vi "To Unix Time.vi"(0 "timestamp":timestamp) -> (2 "unix time":u32)   [LabVIEW 2013, in "libssh2.lvlib"]
doc: "Convert a LabVIEW timestamp to Unix time."
uses:
  libssh2.lvlib
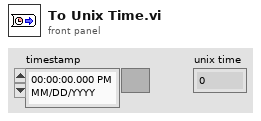
[diagram p1: front panel]
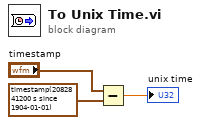
[diagram p0: block diagram]
diagram:
  n1 = Subtract(x="timestamp", y=timestamp(2082841200 s since 1904-01-01)) -> (x-y=→"unix time":dbl)
